vi "ReadXML_TCP.vi"(3 "error in":errorcluster, 4 "timeout ms (3000)":i32=3000, 5 "connection ID in":refnum<k5>) -> (0 "error out":errorcluster, 1 "data out":string, 2 "connection ID out":refnum<k5>)   [LabVIEW 2013]
panel:
  out "String":string
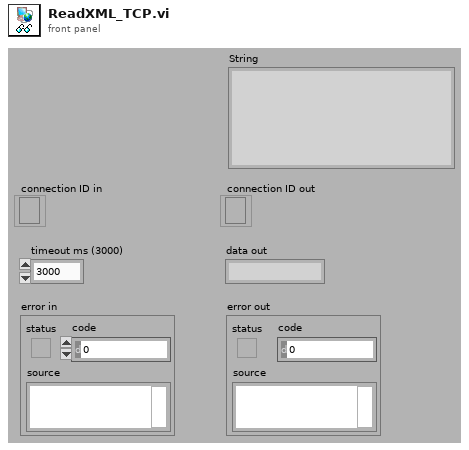
[diagram p1: front panel]
types:
  T1 = enum16{"Standard", "Buffered", "CRLF", "Immediate"}
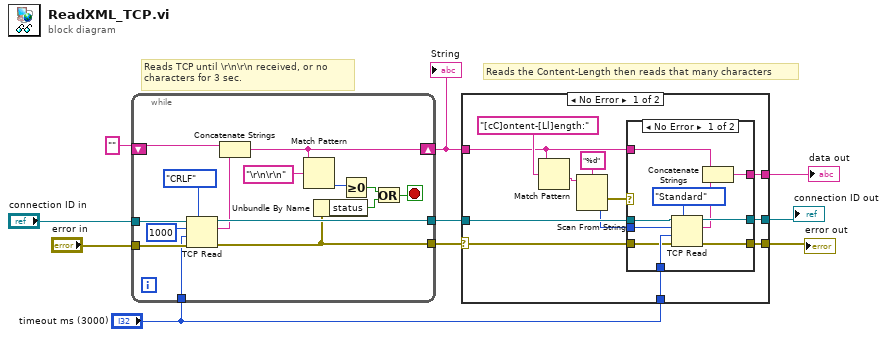
[diagram p0: block diagram]
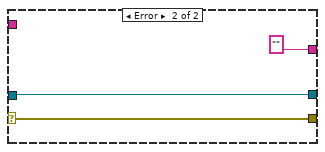
[diagram p3: hidden frame]
diagram:
  # "Reads the Content-Length then reads that many characters"
  # "Reads TCP until \\r\\n\\r\\n received, or no\ncharacters for 3 sec."
  n1 = while {
    tunnel: [w25] -> w6
    tunnel: "connection ID in" -> [w24]
    tunnel: "error in" -> [w23]
    tunnel: [w11] -> w1
    shift-right: [w18] -> w5
    shift-left: "" -> [w19]
    tunnel: "timeout ms (3000)" -> [w12]
    stop <- w13 stop-if-true
    n2 = TCP Read(connection ID=w24, bytes to read=1000, error in (no error)=w23, 7:T1."CRLF" ("mode (standard)"), 9:w12) -> (connection ID out=w25:refnum<k5>, data out=w20:string, error out=w11:errorcluster)
    n3 = Concatenate Strings(w19, w20) -> (w18:string)
    n4 = Match Pattern(string=w18, regular expression="\r\n\r\n") -> (offset past match=w16:i32)  [unwired: 1 in, 3 out]
    n5 = Unbundle By Name(w11) -> ("status"=w14:bool)
    n6 = Greater Or Equal To 0?(x=w16) -> (x >= 0?=w15:bool)
    n7 = Or(x=w15, y=w14) -> (x .or. y?=w13:bool)
  }
  "String" <- w5
  n8 = case shown="No Error" w1 {
    selector: w1 -> [w26 w51]
    tunnel: "timeout ms (3000)" -> [w37 _]
    tunnel: [w28 "" ("data out")] -> w9
    tunnel: [w36 w53] -> w8
    tunnel: [w35 w51] -> w7
    tunnel: w6 -> [w34 w53]
    tunnel: w5 -> [w29 _]
    frame No Error {
      n9 = Match Pattern(string=w29, regular expression="[cC]ontent-[Ll]ength:") -> (after substring=w31:string)  [unwired: 1 in, 3 out]
      n10 = Scan From String(format string="%d", input string=w31) -> (error out=w27:errorcluster, output 1=w33:i32)  [unwired: 3 in, 2 out]
      n11 = case shown="No Error" w27 {
        tunnel: w37 -> [w47 _]
        tunnel: [w46 w48] -> w36
        tunnel: [w45 w49] -> w35
        tunnel: w26 -> [w44 w49]
        tunnel: w34 -> [w43 w48]
        tunnel: w33 -> [w41 _]
        tunnel: w29 -> [w40 w50]
        tunnel: [w38 w50] -> w28
        frame No Error {
          n12 = TCP Read(connection ID=w43, bytes to read=w41, error in (no error)=w44, 7:T1."Standard" ("mode (standard)"), 9:w47) -> (connection ID out=w46:refnum<k5>, data out=w39:string, error out=w45:errorcluster)
          n13 = Concatenate Strings(w40, w39) -> (w38:string)
        }
        frame Error {
        }
      }
    }
    frame Error {
    }
  }
  "data out" <- w9
  "connection ID out" <- w8
  "error out" <- w7
